vi "GEM_BANK_Read_Bank_Counter.vi"(8 "error in (no error)":errorcluster, 11 "GEM_BANK_ARRAY in":refnum<class "GEM_BANK_ARRAY.lvclass">) -> (0 "error out":errorcluster, 2 "Bank Counter":u32, 3 "GEM_BANK_ARRAY out":refnum<class "GEM_BANK_ARRAY.lvclass">)   [LabVIEW 2018, in "GEM_BANK_ARRAY.lvclass"]
uses:
  GEM_BANK_ARRAY.lvclass
  GEM_BANK_ARRAY.lvclass/GEM_BANK_ARRAY.ctl
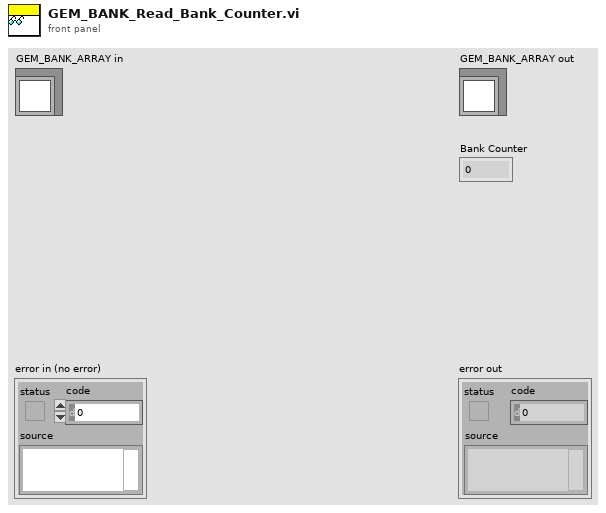
[diagram p1: front panel]
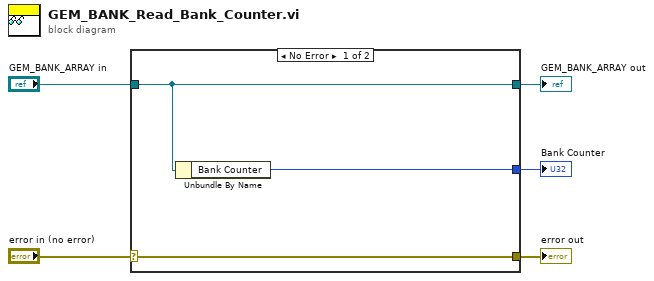
[diagram p0: block diagram]
diagram:
  n1 = case shown="No Error" "error in (no error)" {
    selector: "error in (no error)" -> [w8 w9]
    tunnel: [w8 w9] -> w4
    tunnel: [w7 w10] -> w2
    tunnel: "GEM_BANK_ARRAY in" -> [w7 w10]
    tunnel: [w6 _] -> w1
    frame No Error {
      n2 = Unbundle By Name(w7) -> ("Bank Counter"=w6:u32)
    }
    frame Error {
    }
  }
  "error out" <- w4
  "GEM_BANK_ARRAY out" <- w2
  "Bank Counter" <- w1
